vi "Check_Type_of_PR-dot-1.vi"(1 "[IN] dot status":i16) -> (0 "[OUT] Type of\nproblem dot":i32)   [LabVIEW 2013]
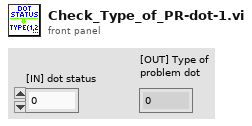
[diagram p1: front panel]
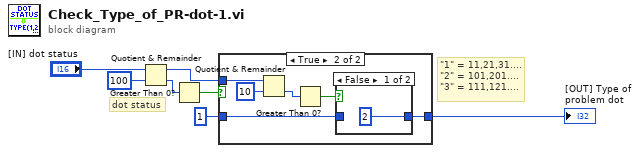
[diagram p0: block diagram]
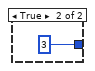
[diagram p3: hidden frame]
diagram:
  # "\"1\" = 11,21,31....\n\"2\" = 101,201....\n\"3\" = 111,121...."
  # "dot status"
  n1 = Quotient & Remainder(x="[IN] dot status", y=i16 100) -> (x-y*floor(x/y)=w7:i16, floor(x/y)=w4:i16)
  n2 = Greater Than 0?(x=w4) -> (x > 0?=w5:bool)
  n3 = case shown="True" w5 {
    tunnel: 1 -> [w8 w10]
    tunnel: w7 -> [_ w14]
    tunnel: [w8 w9] -> w1
    frame False {
    }
    frame True {
      n4 = Quotient & Remainder(x=w14, y=i16 10) -> (floor(x/y)=w12:i16)  [unwired: 1 out]
      n5 = Greater Than 0?(x=w12) -> (x > 0?=w11:bool)
      n6 = case shown="False" w11 {
        tunnel: w10 -> [_ _]
        tunnel: [2 3] -> w9
        frame False {
        }
        frame True {
        }
      }
    }
  }
  "[OUT] Type of\nproblem dot" <- w1
